vi "mkdir.vi"(8 "error in (no error)":errorcluster) -> (0 "error out":errorcluster, 3 "created path":path)   [LabVIEW 2018, in "Application.lvlib"]
uses:
  Application.lvlib
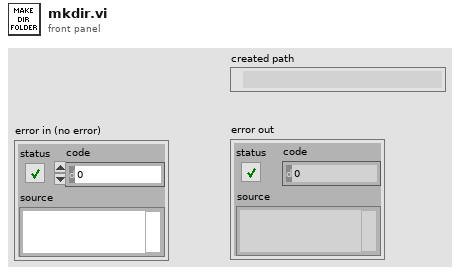
[diagram p1: front panel]
types:
  T1 = typedef "LVDateTimeRec.ctl" = cluster{"fractional second":dbl, "second":i32, "minute":i32, "hour":i32, "day of month":i32, "month":i32, "year":i32, "day of week":i32, "day of year":i32, "DST":i32}
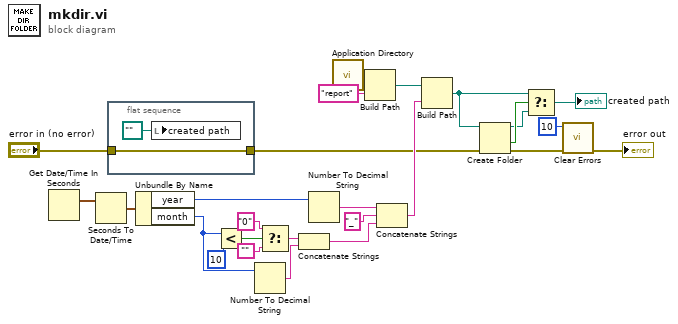
[diagram p0: block diagram]
diagram:
  n1 = Get Date/Time In Seconds() -> (seconds since 1Jan1904=w25:timestamp)
  n2 = Seconds To Date/Time(time stamp (now)=w25) -> (date time rec=w24:T1)  [unwired: 1 in]
  n3 = flat-sequence {
    tunnel: [w27] -> w2
    tunnel: "error in (no error)" -> [w27]
    frame #0 {
      n4 = local write "created path"(path "" ("created path")) -> ()
    }
  }
  n5 = Unbundle By Name(w24) -> ("year"=w23:i32, "month"=w10:i32)
  n6 = Less?(x=w10, y=10) -> (x < y?=w9:bool)
  n7 = Number To Decimal String(number=w10) -> (decimal integer string=w5:string)  [unwired: 1 in]
  n8 = Select(t="0" ("string"), s=w9, f="") -> (s? t:f=w6:string)
  n9 = Concatenate Strings(w6, w5) -> (w4:string)
  n10 = Number To Decimal String(number=w23) -> (decimal integer string=w22:string)  [unwired: 1 in]
  n11 = call <vilib>:"Application Directory.vi"() -> ("Application Directory"=w20:path)
  n12 = Build Path(base path=w20, name or relative path="report") -> (appended path=w17:path)
  n13 = Concatenate Strings(w22, "_" ("string"), w4) -> (w26:string)
  n14 = Build Path(base path=w17, name or relative path=w26) -> (appended path=w3:path)
  n15 = Create Folder(path (use dialog)=w3, error in=w2) -> (created path=w16:path, cancelled=w18:bool, error out=w13:errorcluster)  [unwired: 1 in]
  n16 = Select(t=w3, s=w18, f=w16) -> (s? t:f=→"created path":path)
  n17 = call <vilib>:"Clear Errors.vi"("error in (no error)"=w13, "specific error code to clear (0: all)"=10) -> ("error out"=→"error out":errorcluster)  [unwired: 4 in, 1 out]
